vi "Add.vi"(0 "LV MDI.lvclass":refnum<class "LV MDI.lvclass">, 5 "Document class":refnum<class "Document.lvclass">, 11 "error in (no error)":errorcluster) -> (4 "LV MDI.lvclass":refnum<class "LV MDI.lvclass">, 6 "Doc UID":string, 15 "error out":errorcluster)   [LabVIEW 2016, in "LV MDI.lvclass"]
doc: "Load Documents into memory"
uses:
  LV MDI.lvclass
  Document/Document base/Document.lvclass
  Document/Document base/Document.lvclass/Document.ctl
  LV MDI.lvclass/LV MDI.ctl
  Document/Document base/property/Read Doc Hwnd.vi
  Document/Document base/property/Read Doc UID.vi
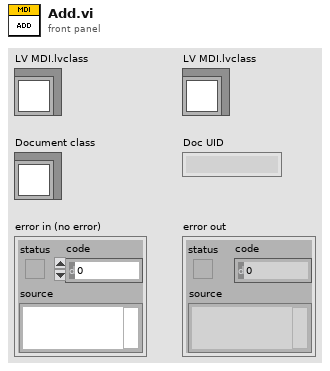
[diagram p1: front panel]
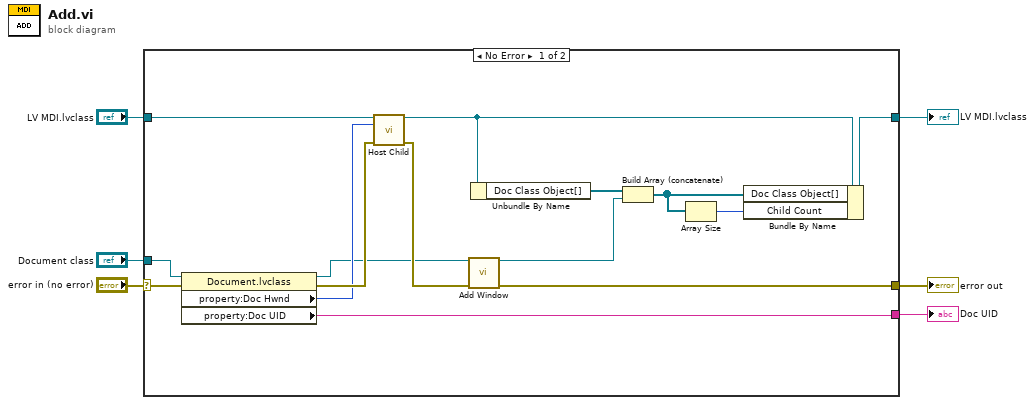
[diagram p0: block diagram]
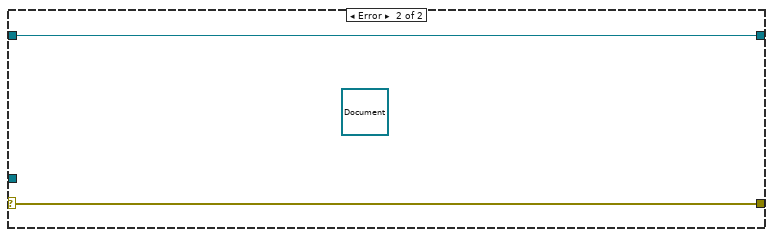
[diagram p2: hidden frame]
diagram:
  n1 = case shown="No Error" "error in (no error)" {
    selector: "error in (no error)" -> [w21 w23]
    tunnel: [w15 w23] -> w5
    tunnel: [w9 w22] -> w3
    tunnel: "LV MDI.lvclass" -> [w13 w22]
    tunnel: "Document class" -> [w20 _]
    tunnel: [w17 _] -> w1
    frame No Error {
      n2 = property class="Document.lvclass"(reference=w20, error in=w21) -> (reference out=w14:refnum<class "Document.lvclass">, error out=w19:errorcluster, "property:Doc Hwnd"=w18:u32, "property:Doc UID"=w17:string)
      n3 = call "Host Child.vi"("LV MDI in"=w13, "Child Hwnd"=w18, "error in (no error)"=w19) -> ("LV MDI out"=w8:refnum<class "LV MDI.lvclass">, "error out"=w16:errorcluster)  [unwired: 11 in]
      n4 = call-dynamic "Add Window.vi"("Document in"=w14, "error in (no error)"=w16) -> ("Document out"=w7:refnum<class "Document.lvclass">, "error out"=w15:errorcluster)  [unwired: 12 in]
      n5 = Unbundle By Name(w8) -> ("Doc Class Object[]"=w12:refnum<class "Document.lvclass">[])
      n6 = Build Array (concatenate)(w12, w7) -> (w11:refnum<class "Document.lvclass">[])
      n7 = Array Size(array=w11) -> (size(s)=w10:i32)
      n8 = Bundle By Name(cluster=w8, "Doc Class Object[]"=w11, "Child Count"=w10) -> (w9:refnum<class "LV MDI.lvclass">)
    }
    frame Error {
      (unwired) refnum<class "Document.lvclass"> refnum ("Document out")
    }
  }
  "error out" <- w5
  "LV MDI.lvclass" <- w3
  "Doc UID" <- w1
